vi "W7X1DJSON.vi"(4 "values":sgl[](array[numeric]), 5 "label":string, 7 "Unit":string, 8 "dimensions":i64[](array[numeric]), 9 "dimensionCount":i32, 11 "datatype":string) -> (3 "JSON string":string)   [LabVIEW 2014]
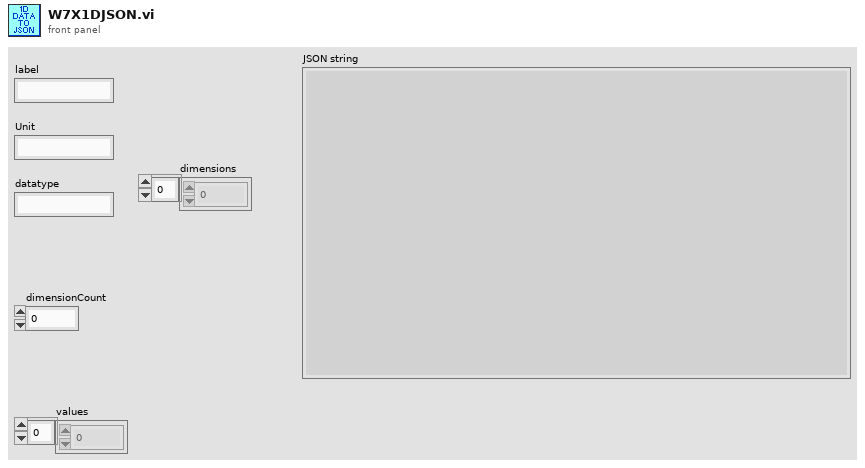
[diagram p1: front panel]
types:
  T1 = cluster{"label":string, "Unit":string, "datatype":string, "dimensionCount":i32, "values":sgl[], "dimensions":i64[]}
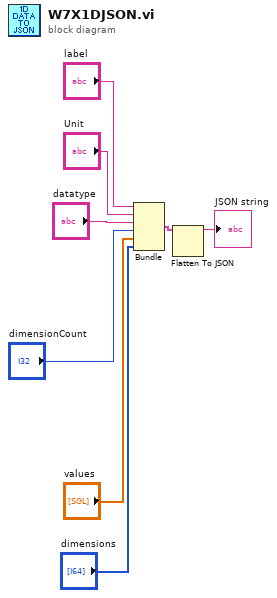
[diagram p0: block diagram]
diagram:
  n1 = Bundle("label"="label", "Unit"="Unit", "datatype"="datatype", "dimensionCount"="dimensionCount", "values"="values", "dimensions"="dimensions") -> (w7:T1)  [unwired: 1 in]
  n2 = Flatten To JSON(anything=w7) -> (JSON string=→"JSON string":string)  [unwired: 2 in, 1 out]
